vi "RESTful Validate Control Type.vi"(10 "Type String":string) -> (2 "Invalid RESTful Type?":bool)   [LabVIEW 2020]
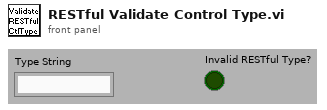
[diagram p1: front panel]
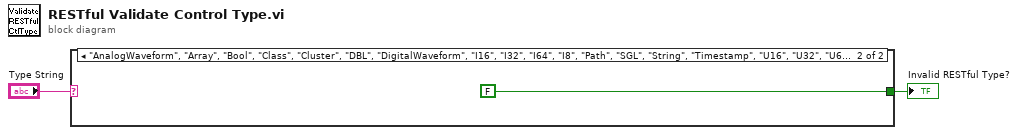
[diagram p0: block diagram]
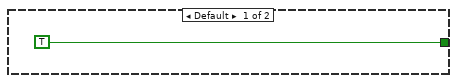
[diagram p2: hidden frame]
diagram:
  n1 = case shown="\"AnalogWaveform\", \"Array\", \"Bool\", \"Class\", \"Cluster\", \"DBL\", \"DigitalWaveform\", \"I16\", \"I32\", \"I64\", \"I8\", \"Path\", \"SGL\", \"String\", \"Timestamp\", \"U16\", \"U32\", \"U64\", \"U8\"" "Type String" {
    tunnel: [TRUE ("Is Valid RESTful Type?") FALSE ("Is Valid RESTful Type?")] -> w1
    frame Default {
    }
    frame "AnalogWaveform", "Array", "Bool", "Class", "Cluster", "DBL", "DigitalWaveform", "I16", "I32", "I64", "I8", "Path", "SGL", "String", "Timestamp", "U16", "U32", "U64", "U8" {
    }
  }
  "Invalid RESTful Type?" <- w1
